vi "case_structure.vi"() -> ()   [LabVIEW 2020]
panel:
  in  "Enum":enum16{"Jeff", "Stephanie", "John"}(ring)=enum."John"
  out "Height":dbl
  # "Height Demo"
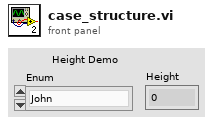
[diagram p1: front panel]
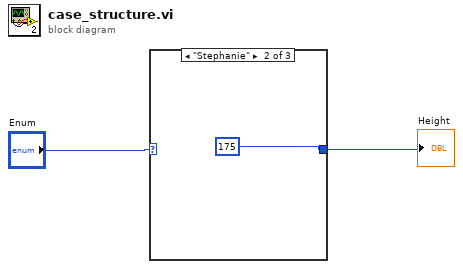
[diagram p0: block diagram]
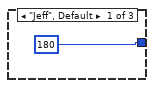
[diagram p2: hidden frame]
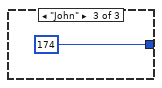
[diagram p3: hidden frame]
diagram:
  n1 = case shown="\"Stephanie\"" "Enum" {
    tunnel: [180 175 174] -> w1
    frame "Jeff", Default {
    }
    frame "Stephanie" {
    }
    frame "John" {
    }
  }
  "Height" <- w1
